vi "Host Image Acquisition Module.vi"(8 "error in":errorcluster, 11 "Operation":T3) -> (0 "error out":errorcluster, 1 "Image Acquired":bool, 2 "Acq In Progress":bool, 3 "Image":T2(plugin-control))   [LabVIEW 2013]
uses:
  Host Image Acquisition Module Enum.ctl
  Acquisition Settings Cluster.ctl
  <vilib>/vision/Image Controls.llb/IMAQ Image.ctl
  Image Acquisition Settings FG Enum.ctl
  System Status/Status FG Enum.ctl
  Image Processing/Mask ROI FG Enum.ctl
  <vilib>/rvi/interface/RandomDataEmulation/niFpgaWriteControlTemplate.vi
  <vilib>/rvi/interface/RandomDataEmulation/nirviRandomDataRunMethod.vi
  <vilib>/rvi/interface/RandomDataEmulation/nirviRandomDataDMAMethods.vi
  <vilib>/rvi/interface/RandomDataEmulation/niFpgaReadControlTemplate.vi
  Globals/Average Sector Data.vi
  <vilib>/rvi/interface/RandomDataEmulation/nirviRandomDataClose.vi
  <vilib>/rvi/interface/nirviReadWriteControl/nirviReadWriteControl.xnode
  FGs/FPGA_Reference.ctl
  Common/CL Configuration.ctl
  Common/CL Signal Mapping.ctl
  10-Tap 8-bit Camera without DRAM (FPGA-SIM).vi
  <vilib>/rvi/interface/nirviMethod/nirviMethod.xnode
  FPGA/Sector/Accumulate/Sector Parameter Cluster.ctl
  <vilib>/rvi/interface/nirviCloseFPGA/nirviCloseFPGA.xnode
  Common/Timing/Timing Lib.lvlib
  <vilib>/rvi/errors/niLvFpgaMergeErrorWithErrorCode.vi
panel:
  out "Actual Depth":u32
  out "Target Sim TO":bool
  out "Cam Data Timeout":bool
  out "Sector FIFO Timeout":bool
  out "Host DMA Timeout":bool
  out "Number of Elements to Write Host DMA":u32
  out "Number of Elements to Read Cam Data":u32
  out "Image Data":u64[](array[numeric])
  out "Elements Remaining":u32
  out "Words per image":u32
  out "Num Frames read":u32
  out "DMA Words per Image":u32
  out "Acquire":bool
  in  "Acquisition Settings Cluster":T1={"Image Width"=2040, "Image Height"=1088, "Frames To Acquire"=0, "Signal Mapping"=enum."Basler 10-tap", "DMA Buffer Size\n(In Images)"=64} {"Image Height" max=65535; "Image Width" max=65535 step=40}
  out "Buffer Size":u32
  out "Acq'd Frame Width":u32=2040
  out "DMA Write Timeout":bool
  in  "Start Serial Server":bool
  out "Frames Acq'd":u32=1
  out "Acq'd Frame Height":u32=1088
  out "Initialized":bool
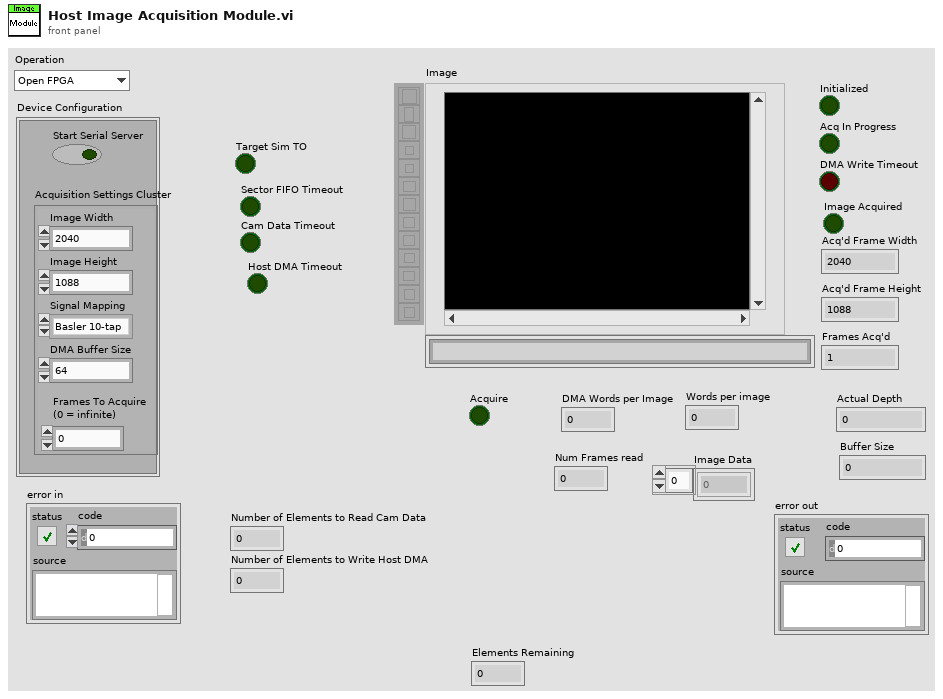
[diagram p1: front panel]
types:
  T1 = typedef "Acquisition Settings Cluster.ctl" = cluster{"Image Width":u32, "Image Height":u32, "Frames To Acquire":u32, "Signal Mapping":enum8{"Standard", "Basler 10-tap", "Vosskühler 10-tap"}, "DMA Buffer Size\n(In Images)":u32}
  T2 = typedef "IMAQ Image.ctl" = refnum<image>
  T3 = typedef "Host Image Acquisition Module Enum.ctl" = enum16{"Open FPGA", "Initialize DMA FIFO", "Load Sim Images", "Initialize Acquisition", "Update Sector Parameters", "Start Acquisition", "Aquire Image", "Read Averages", "Cancel Acquisition", "Close FPGA"}
  T4 = enum8{"Standard", "Basler 10-tap", "Vosskühler 10-tap"}
  T5 = typedef "Image Acquisition Settings FG Enum.ctl" = enum16{"Read", "Write"}
  T6 = typedef "Status FG Enum.ctl" = enum16{"Reset", "Read", "Write"}
  T7 = typedef "Mask ROI FG Enum.ctl" = enum16{"Read", "Write"}
  T8 = enum16{"big-endian, network order", "native, host order", "little-endian"}
  T9 = typedef "FPGA_Reference.ctl" = refnum<k20>
  T10 = typedef "Image Type" = u32
  T11 = typedef "Mask ROI Cluster.ctl" = cluster{"left annulus":T12, "right annulus":T12, "Threshold Range":cluster{"Lower value":dbl, "Upper value":dbl}, "[Avg BG]":u8[], "Number of Sectors":u8, "Left ROI":T13, "Right ROI":T13, "Left Start Angle Duty Cycle":fxp<+,8,0>, "Left End Angle Duty Cycle":fxp<+,8,0>, "Right End Angle Duty Cycle":fxp<+,8,0>, "Right Start Angle Duty Cycle":fxp<+,8,0>, "[Sector ROIs]":T13[]}
  T12 = typedef "IMAQ Circle" = cluster{"Center X":i32, "Center Y":i32, "Inner Radius":i32, "Outer Radius":i32, "Start Angle":dbl, "End Angle":dbl}
  T13 = typedef "ROI Descriptor" = cluster{"Global Rectangle":i32[], "Contours":cluster{"ID":enum32{"External", "Internal"}, "Type":u32, "Coordinates":i32[]}[]}
  T14 = typedef "Sector Parameter Cluster.ctl" = cluster{"Start Angle":fxp<+/-,17,2>, "End Angle":fxp<+,17,3>, "Inner Radius":u16, "Outter Radius":u16, "Hinge X":u16, "Hinge Y":u16, "NumWingSectors":u8}
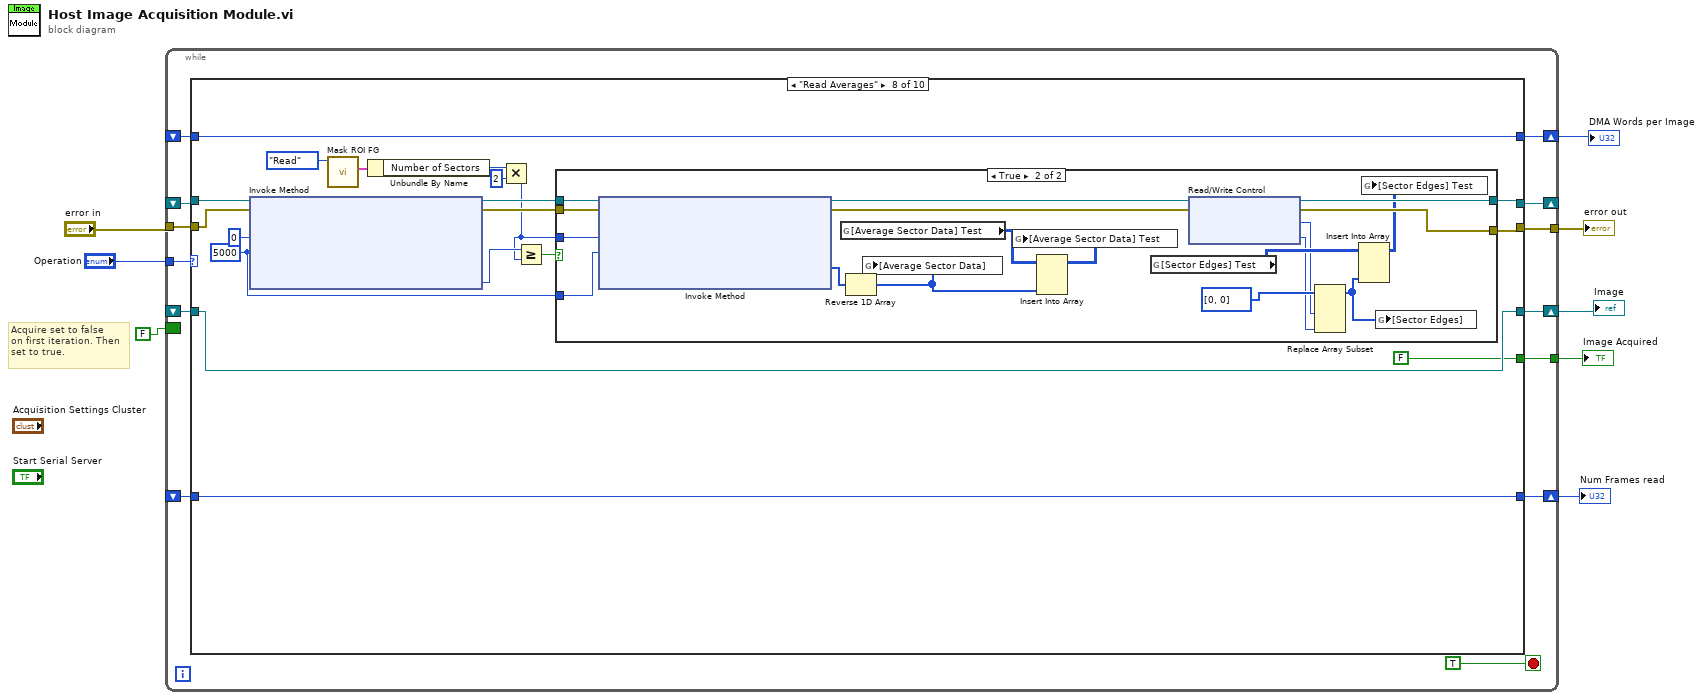
[diagram p0: block diagram]
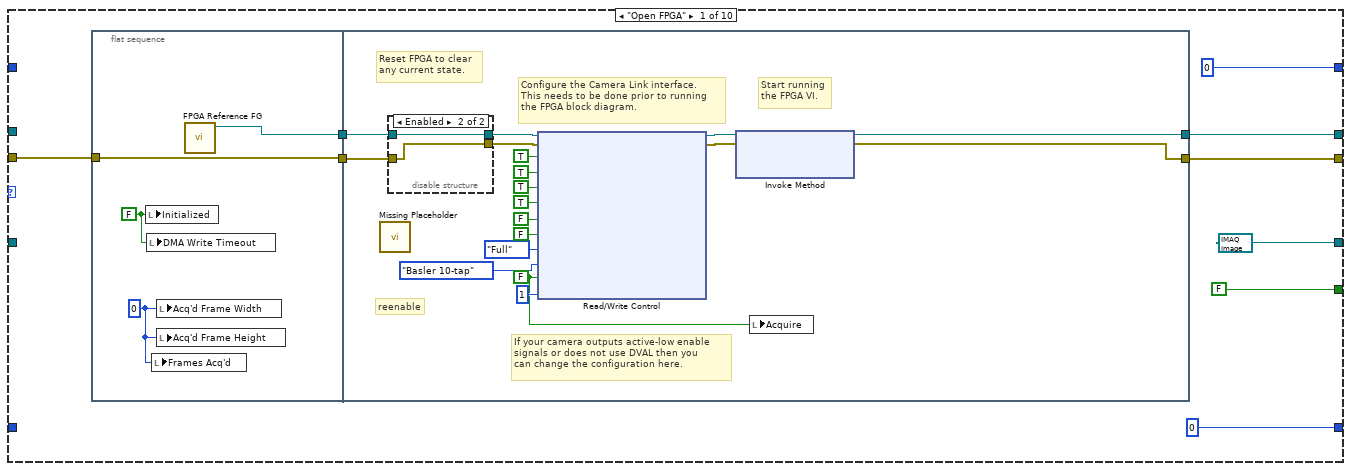
[diagram p2: hidden frame]
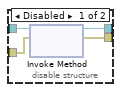
[diagram p3: hidden frame]
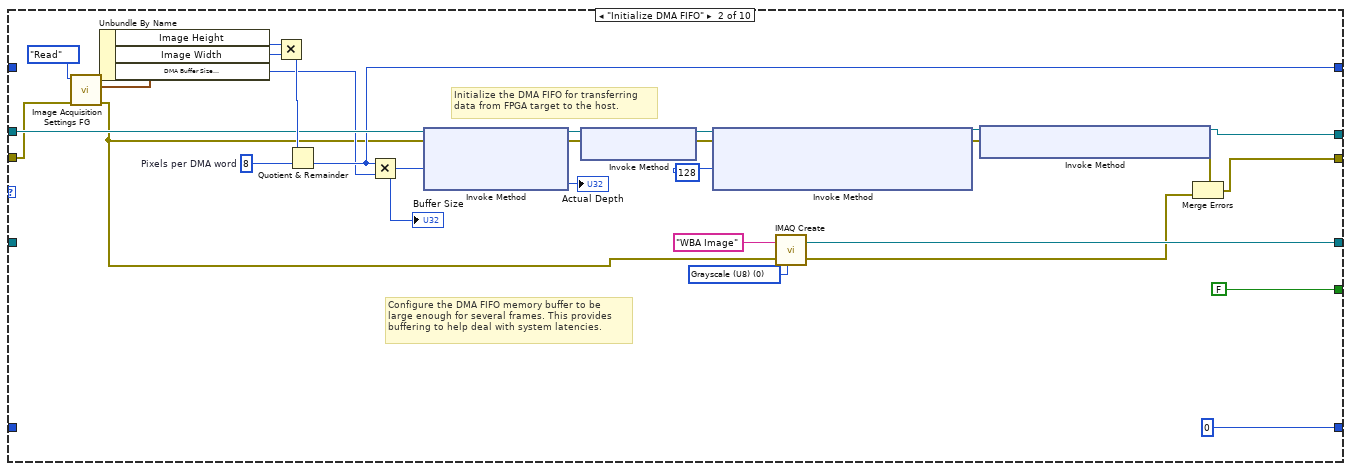
[diagram p4: hidden frame]
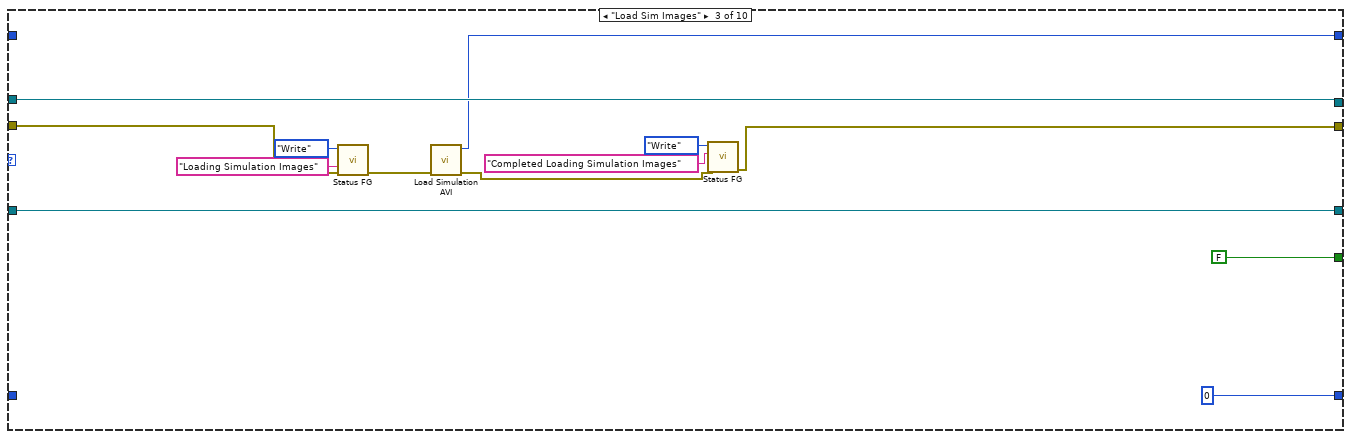
[diagram p5: hidden frame]
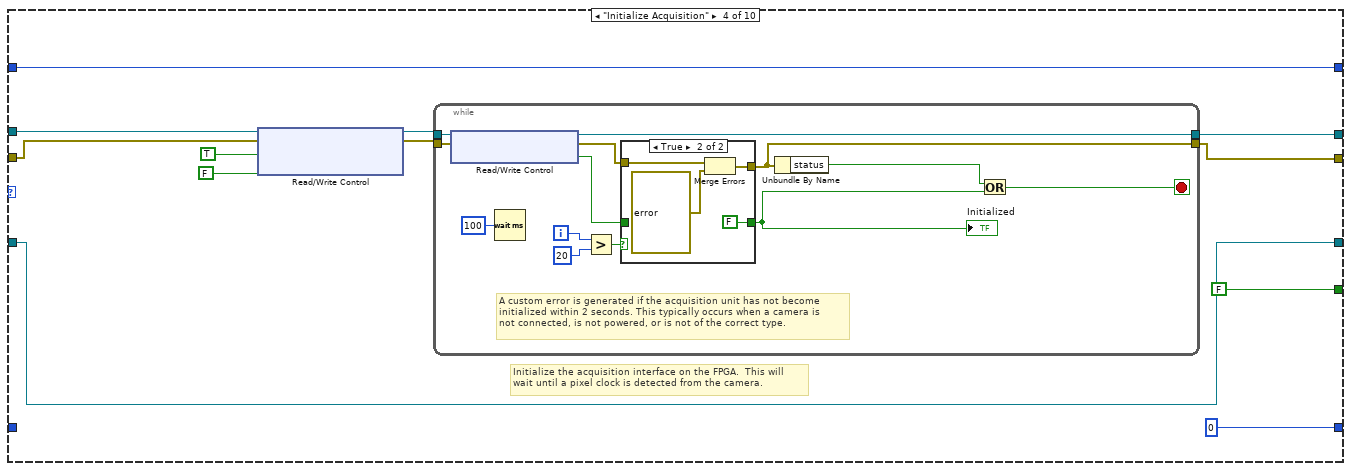
[diagram p6: hidden frame]
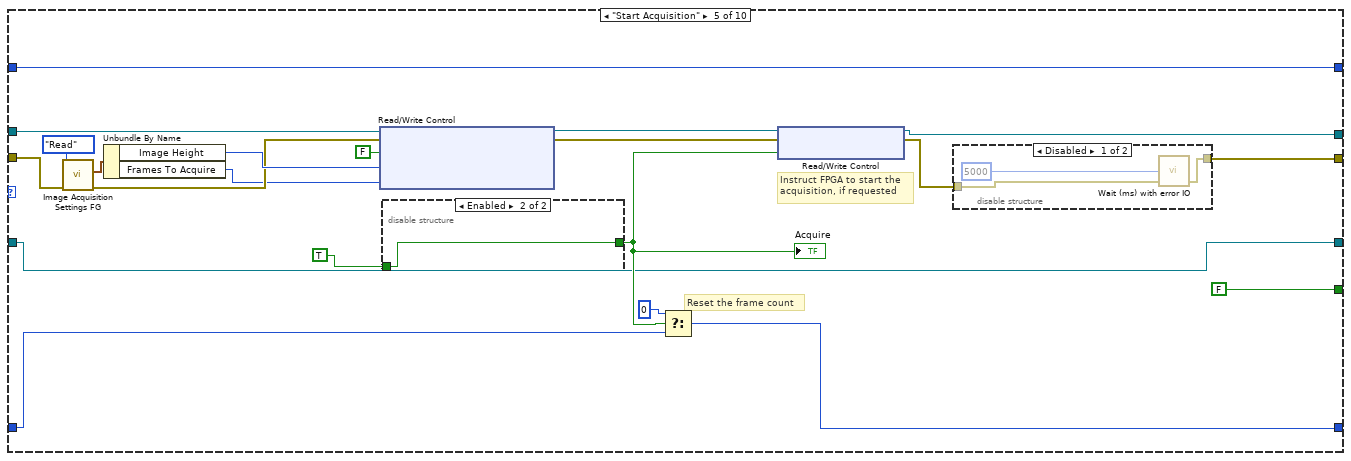
[diagram p8: hidden frame]
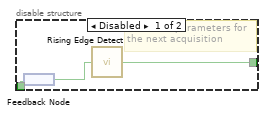
[diagram p10: hidden frame]
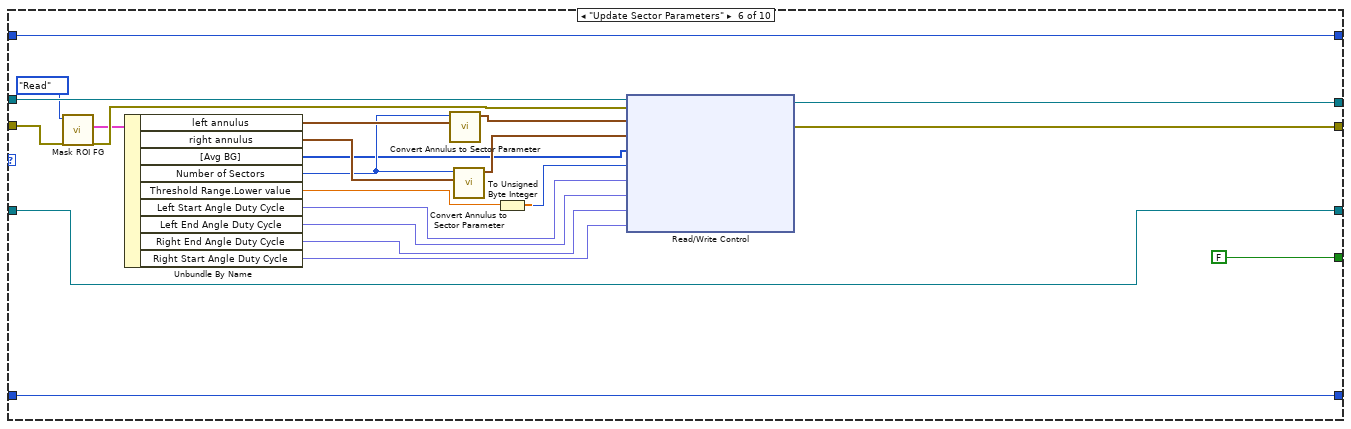
[diagram p11: hidden frame]
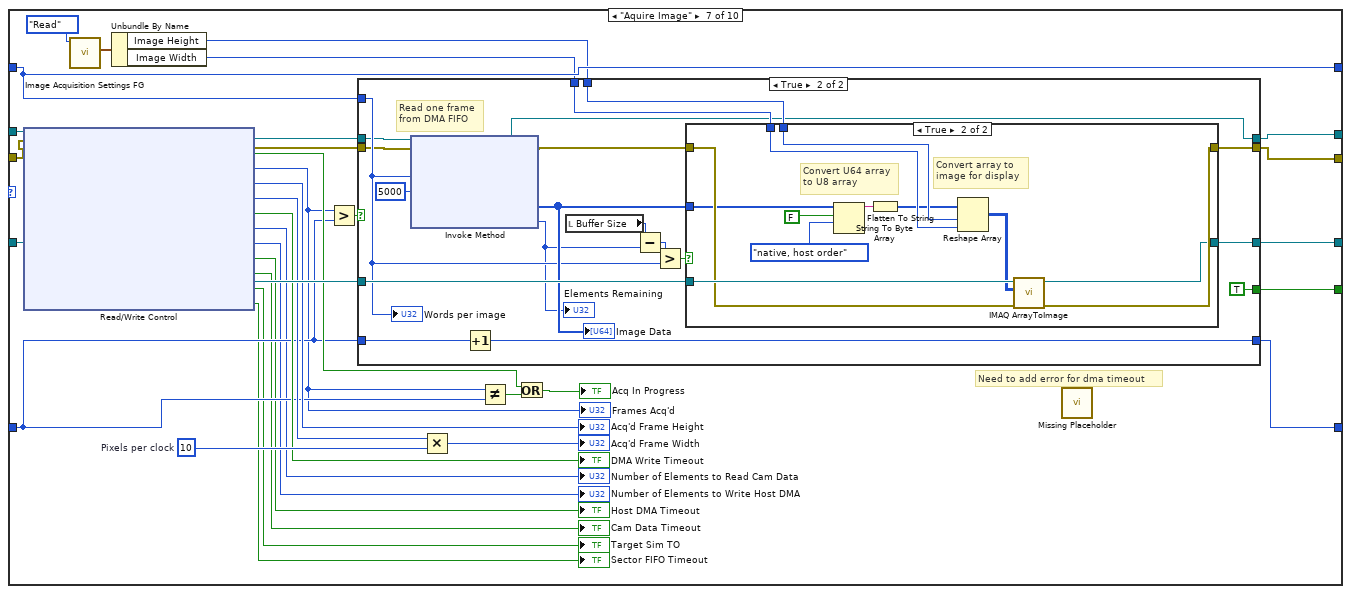
[diagram p12: hidden frame]
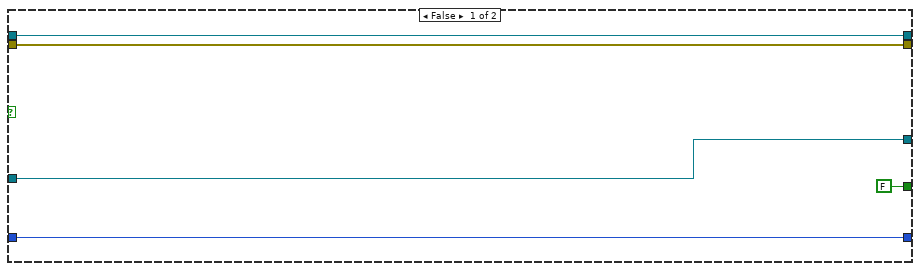
[diagram p13: hidden frame]
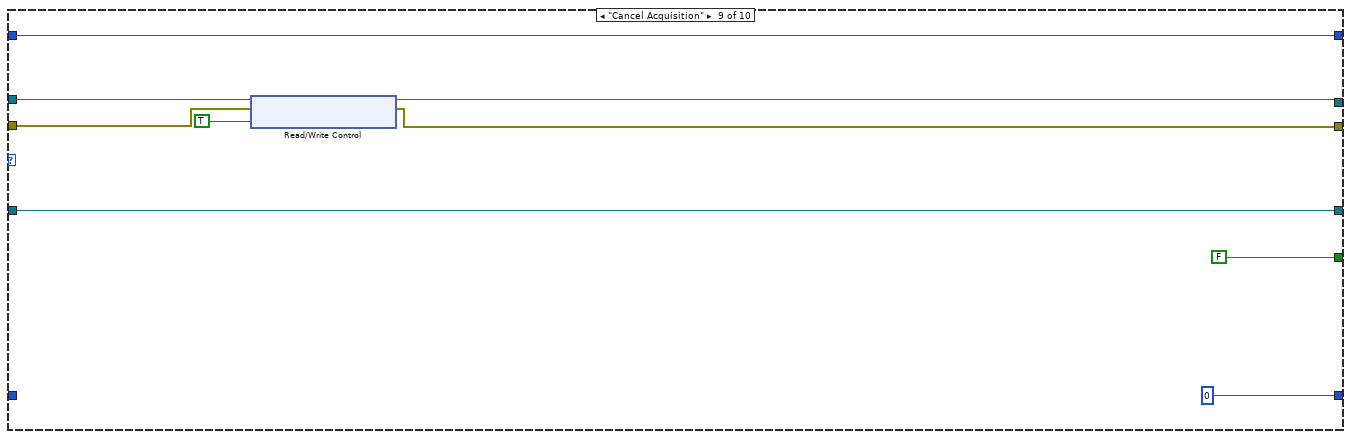
[diagram p16: hidden frame]
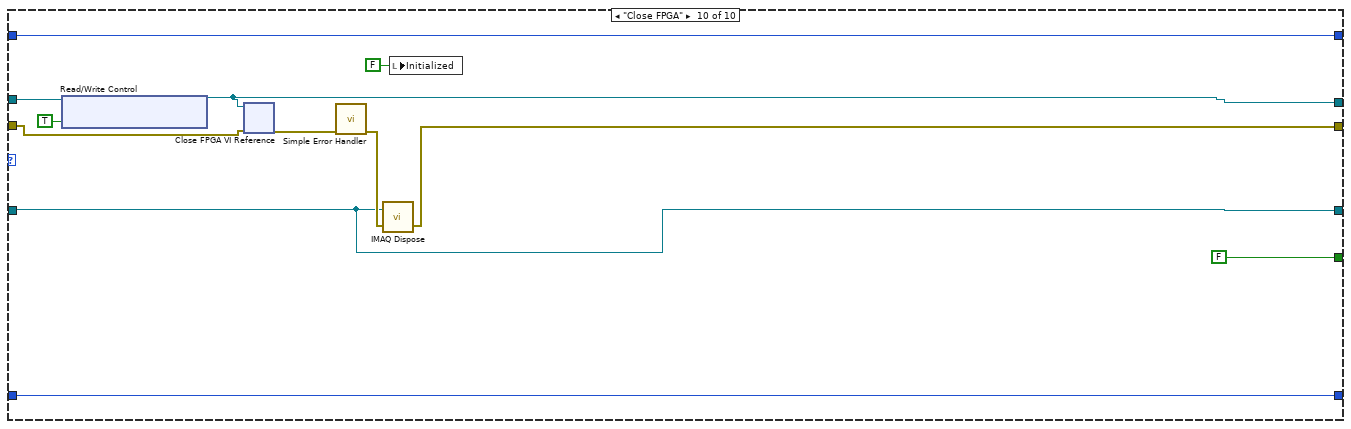
[diagram p17: hidden frame]
diagram:
  # "Acquire set to false\non first iteration. Then\nset to true."
  n1 = while {
    shift-right: [w20] -> _
    shift-left: _ -> [w16]
    tunnel: "error in" -> [w19]
    tunnel: "Operation" -> [w18]
    tunnel: [w17] -> w6
    shift-right: [w15] -> w3
    shift-left: _ -> [w14]
    shift-right: [w13] -> w4
    shift-left: _ -> [w10]
    shift-right: [w12] -> w2
    shift-left: _ -> [w11]
    border: FALSE ("Acquire") -> [_]
    tunnel: [w9] -> w1
    stop <- TRUE stop-if-true
    n2 = case shown="\"Read Averages\"" w18 {
      tunnel: w19 -> [w30 w74 w95 w102 w145 w181 w196 w265 w297 w303]
      tunnel: [w29 w66 w98 w108 w138 w177 w214 w271 w299 w304] -> w20
      tunnel: [w28 w67 w89 w104 w136 w178 w213 w266 w296 w310] -> w17
      tunnel: w16 -> [_ w82 w98 w109 w146 w183 w215 w272 w301 w306]
      tunnel: [u32 0 w81 w97 w107 w141 w182 w206 w270 w295 w307] -> w15
      tunnel: w14 -> [_ _ _ w107 w141 w182 w206 w270 w295 w307]
      tunnel: [T2 refnum ("New Image") w77 w99 w103 w140 w168 w208 w269 w298 w308] -> w13
      tunnel: [u32 0 u32 0 u32 0 u32 0 w142 w176 w212 w268 u32 0 w309] -> w12
      tunnel: w11 -> [_ _ _ _ w143 w176 w194 w268 _ w309]
      tunnel: w10 -> [_ _ w99 w103 w140 w168 w207 w269 w298 w308]
      tunnel: [FALSE ("Image Acquired") FALSE ("Image Acquired") FALSE ("Image Acquired") FALSE ("Image Acquired") FALSE ("Image Acquired") FALSE ("Image Acquired") w188 FALSE ("Image Acquired") FALSE ("Image Acquired") FALSE ("Image Acquired")] -> w9
      frame "Open FPGA" {
        n3 = flat-sequence {
          tunnel: w30 -> [w31]
          tunnel: [w32] -> w27
          tunnel: [w31] -> w26
          tunnel: [w37] -> w28
          tunnel: [w38] -> w29
          tunnel: w27 -> [w42]
          tunnel: w26 -> [w39]
          frame #0 {
            w33 = u32 0 ("Acq'd Frame Width")
            w34 = FALSE ("Initialized")
            n4 = local write "Initialized"(w34) -> ()
            n5 = local write "DMA Write Timeout"(w34) -> ()
            n6 = local write "Frames Acq'd"(w33) -> ()
            n7 = local write "Acq'd Frame Width"(w33) -> ()
            n8 = local write "Acq'd Frame Height"(w33) -> ()
            n9 = call "FPGA Reference FG.vi"() -> ("FPGA VI Reference Out"=w32:T9)  [unwired: 11 in]
          }
          frame #1 {
            w35 = FALSE ("Acq Control.Acquire")
            # "reenable"
            # "If your camera outputs active-low enable\nsignals or does not use DVAL then you \ncan change the configuration here."
            # "Start running\nthe FPGA VI."
            # "Reset FPGA to clear\nany current state."
            # "Configure the Camera Link interface.\nThis needs to be done prior to running\nthe FPGA block diagram."
            n10 = call "Missing Placeholder.vi"() -> ()  [unwired: 12 in]
            n11 = disable-structure shown="Enabled" {
              disable-tunnel: [w56 w58] -> w46
              disable-tunnel: [w55 w57] -> w44
              disable-tunnel: w42 -> [w54 w58]
              disable-tunnel: w39 -> [w53 w57]
              frame Disabled {
                n12 = xnode "Invoke Method"("FPGA VI Reference In"=w54, "error in"=w53) -> ("FPGA VI Reference Out"=w56:T9, "error out"=w55:errorcluster)
              }
              frame Enabled {
              }
            }
            n13 = xnode "Read/Write Control"("FPGA VI Reference In"=w46, "error in"=w44, "CL Config.FVAL Active High"=TRUE ("IO Module Config.CL FVAL Active High"), "CL Config.LVAL Active High"=TRUE ("IO Module Config.CL LVAL Active High"), "CL Config.DVAL Active High"=TRUE ("IO Module Config.CL DVAL Active High"), "CL Config.Spare Active High"=TRUE ("IO Module Config.CL Spare Active High"), "CL Config.Line Scan"=FALSE, "Acq Control.Ignore DVAL"=FALSE ("CL Config.Line Scan"), "CL Config.Configuration"=enum8{"Base", "Medium", "Full"}."Full", "CL Config.Signal Mapping"=T4."Basler 10-tap", "Acq Control.Acquire"=w35, "# of Frames to Average"=u8 1) -> ("FPGA VI Reference Out"=w43:T9, "error out"=w45:errorcluster)
            n14 = xnode "Invoke Method"("FPGA VI Reference In"=w43, "error in"=w45) -> ("FPGA VI Reference Out"=w38:T9, "error out"=w37:errorcluster)  [unwired: 1 in]
            n15 = local write "Acquire"(w35) -> ()
          }
        }
      }
      frame "Initialize DMA FIFO" {
        w78 = T10 0 items=["Grayscale (U8)", "Grayscale (I16)", "Grayscale (SGL)", "Complex (CSG)", "RGB (U32)", "HSL (U32)", "RGB (U64)", "Grayscale (U16)"] ("Image Type")
        w84 = u32 8  # Pixels per DMA word
        # "Configure the DMA FIFO memory buffer to be\nlarge enough for several frames. This provides\nbuffering to help deal with system latencies."
        # "Initialize the DMA FIFO for transferring\ndata from FPGA target to the host."
        n16 = call "Image Acquisition Settings FG.vi"("error in (no error)"=w74, "Operation"=Image_Acquisition_Settings_FG_Enum."Read") -> ("error out"=w69:errorcluster, "Acquisition Settings Out"=w75:T1)  [unwired: 8 in]
        n17 = Unbundle By Name(w75) -> ("Image Height"=w73:u32, "Image Width"=w72:u32, "DMA Buffer Size\n(In Images)"=w71:u32)
        n18 = Multiply(x=w73, y=w72) -> (x*y=w83:u32)
        n19 = Quotient & Remainder(x=w83, y=w84) -> (floor(x/y)=w81:u32)  [unwired: 1 out]
        n20 = Multiply(x=w81, y=w71) -> (x*y=w85:u32)
        "Buffer Size" <- w85
        n21 = xnode "Invoke Method"("FPGA VI Reference In"=w82, "error in"=w69, "Requested Depth"=w85) -> ("FPGA VI Reference Out"=w87:T9, "error out"=w86:errorcluster, "Actual Depth"=→"Actual Depth":u32)
        n22 = xnode "Invoke Method"("FPGA VI Reference In"=w87, "error in"=w86) -> ("FPGA VI Reference Out"=w64:T9, "error out"=w62:errorcluster)
        n23 = xnode "Invoke Method"("FPGA VI Reference In"=w64, "error in"=w62, "Requested Depth"=u32 128) -> ("FPGA VI Reference Out"=w61:T9, "error out"=w60:errorcluster)  [unwired: 1 out]
        n24 = call "IMAQ Create"("Image Name"="WBA Image", "Image Type"=w78, "error in (no error)"=w69) -> ("New Image"=w77:T2, "error out"=w68:errorcluster)  [unwired: 2 in]
        n25 = xnode "Invoke Method"("FPGA VI Reference In"=w61, "error in"=w60) -> ("FPGA VI Reference Out"=w66:T9, "error out"=w59:errorcluster)
        n26 = Merge Errors(w59, w68) -> (w67:errorcluster)
      }
      frame "Load Sim Images" {
        n27 = call "Status FG.vi"("error in (no error)"=w95, "Status In"="Loading Simulation Images", "Operation"=Status_FG_Enum."Write") -> ("error out"=w94:errorcluster)  [unwired: 7 in, 1 out]
        n28 = call "Load Simulation AVI.vi"("error in (no error)"=w94) -> ("error out"=w90:errorcluster, "Words per image"=w97:u32)  [unwired: 9 in]
        n29 = call "Status FG.vi"("error in (no error)"=w90, "Status In"="Completed Loading Simulation Images", "Operation"=Status_FG_Enum."Write") -> ("error out"=w89:errorcluster)  [unwired: 7 in, 1 out]
      }
      frame "Initialize Acquisition" {
        # "Initialize the acquisition interface on the FPGA.  This will\nwait until a pixel clock is detected from the camera."
        n30 = xnode "Read/Write Control"("FPGA VI Reference In"=w109, "error in"=w102, "Acq Control.Initialize"=TRUE ("Arm Acquisition"), "Acq Control.Cancel Acq"=FALSE) -> ("FPGA VI Reference Out"=w112:T9, "error out"=w111:errorcluster)
        n31 = while {
          tunnel: w112 -> [w121]
          tunnel: w111 -> [w120]
          tunnel: [w119] -> w108
          tunnel: [w122] -> w104
          i -> [w115]
          stop <- w125 stop-if-true
          # "A custom error is generated if the acquisition unit has not become\ninitialized within 2 seconds. This typically occurs when a camera is\nnot connected, is not powered, or is not of the correct type."
          n32 = xnode "Read/Write Control"("FPGA VI Reference In"=w121, "error in"=w120) -> ("FPGA VI Reference Out"=w119:T9, "error out"=w118:errorcluster, "Acq Status.Initialized"=w117:bool)
          n33 = Wait (ms)(milliseconds to wait=u32 100) -> ()  [unwired: 1 out]
          n34 = Greater?(x=w115, y=20) -> (0:w116:bool)
          n35 = case shown="True" w116 {
            tunnel: [w127 FALSE] -> w113
            tunnel: w117 -> [w127 _]
            tunnel: w118 -> [w126 w129]
            tunnel: [w126 w131] -> w122
            frame False {
            }
            frame True {
              n36 = Merge Errors(w129, errorcluster {"status"=TRUE, "code"=-8999, "source"="Acquisition Initialization: This error typically occurs when a camera is not properly connected, is not powered, or is not of the correct type."} ("error in")) -> (w131:errorcluster)
            }
          }
          "Initialized" <- w113
          n37 = Unbundle By Name(w122) -> ("status"=w124:bool)
          n38 = Or(x=w124, y=w113) -> (x .or. y?=w125:bool)
        }
      }
      frame "Start Acquisition" {
        # "Reset the frame count"
        # "Instruct FPGA to start the\nacquisition, if requested"
        n39 = call "Image Acquisition Settings FG.vi"("error in (no error)"=w145, "Operation"=Image_Acquisition_Settings_FG_Enum."Read") -> ("error out"=w144:errorcluster, "Acquisition Settings Out"=w152:T1)  [unwired: 8 in]
        n40 = Unbundle By Name(w152) -> ("Image Height"=w147:u32, "Frames To Acquire"=w134:u32)
        n41 = xnode "Read/Write Control"("FPGA VI Reference In"=w146, "error in"=w144, "Acq Control.Cancel Acq"=FALSE, "Acq Control.Line Scan Height"=w147, "Acq Control.Frames To Acq"=w134) -> ("FPGA VI Reference Out"=w132:T9, "error out"=w133:errorcluster)
        n42 = disable-structure shown="Enabled" {
          disable-tunnel: [w159 w160] -> w149
          disable-tunnel: TRUE ("Acquire") -> [w157 w160]
          frame Disabled {
            # "Write the parameters for\nthe next acquisition"
            n43 = feedback #1() -> (w158:bool)
            n44 = feedback-in #1(w157) -> ()
            n45 = call "Rising Edge Detect.vi"("Input"=w158) -> ("Pulse"=w159:bool)  [unwired: 4 in]
          }
          frame Enabled {
          }
        }
        "Acquire" <- w149
        n46 = Select(t=u32 0, s=w149, f=w143) -> (s? t:f=w142:u32)
        n47 = xnode "Read/Write Control"("FPGA VI Reference In"=w132, "error in"=w133, "Acq Control.Acquire"=w149) -> ("FPGA VI Reference Out"=w138:T9, "error out"=w137:errorcluster)
        n48 = disable-structure shown="Disabled" {
          disable-tunnel: w137 -> [w154 w156]
          disable-tunnel: [w153 w156] -> w136
          frame Disabled {
            n49 = call "Wait (ms) with error IO.vi"("error in (no error)"=w154, "milliseconds to wait"=u32 5000) -> ("error out"=w153:errorcluster)  [unwired: 3 in]
          }
          frame Enabled {
          }
        }
      }
      frame "Update Sector Parameters" {
        n50 = call "Mask ROI FG.vi"("error in (no error)"=w181, "Operation"=Mask_ROI_FG_Enum."Read") -> ("error out"=w180:errorcluster, "Mask ROI Out"=w175:T11)  [unwired: 8 in]
        n51 = Unbundle By Name(w175) -> ("left annulus"=w174:T12, "right annulus"=w172:T12, "[Avg BG]"=w169:u8[], "Number of Sectors"=w171:u8, "Threshold Range.Lower value"=w166:dbl, "Left Start Angle Duty Cycle"=w164:fxp<+,8,0>, "Left End Angle Duty Cycle"=w163:fxp<+,8,0>, "Right End Angle Duty Cycle"=w162:fxp<+,8,0>, "Right Start Angle Duty Cycle"=w161:fxp<+,8,0>)
        n52 = call "Convert Annulus to Sector Parameter.vi"("Annulus"=w174, "NumWingSectors"=w171) -> ("Sector Parameter"=w173:T14)  [unwired: 9 in]
        n53 = call "Convert Annulus to Sector Parameter.vi"("Annulus"=w172, "NumWingSectors"=w171) -> ("Sector Parameter"=w170:T14)  [unwired: 9 in]
        n54 = To Unsigned Byte Integer(number=w166) -> (unsigned 8bit integer=w165:u8)
        n55 = xnode "Read/Write Control"("FPGA VI Reference In"=w183, "error in"=w180, "Sector Parameters Left"=w173, "Sector Parameters Right"=w170, "[Average BG Intensity]"=w169, "Sector Threshold"=w165, "Left Start Angle Duty Cycle"=w164, "Left End Angle Duty Cycle"=w163, "Right End Angle Duty Cycle"=w162, "Right Start Angle Duty Cycle"=w161) -> ("FPGA VI Reference Out"=w177:T9, "error out"=w178:errorcluster)
      }
      frame "Aquire Image" {
        w204 = u32 10  # Pixels per clock
        # "Need to add error for dma timeout"
        n56 = xnode "Read/Write Control"("FPGA VI Reference In"=w215, "error in"=w196) -> ("FPGA VI Reference Out"=w211:T9, "error out"=w210:errorcluster, "Acq Status.Acq In Progress"=w195:bool, "Acq Status.Frames Acq'd"=w193:u32, "Acq Status.Lines Per Frame"=→"Acq'd Frame Height":u32, "Acq Status.Clocks Per Line"=w203:u32, "Acq Status.DMA Write Timeout"=→"DMA Write Timeout":bool, "Number of Elements to Read Cam Data"=→"Number of Elements to Read Cam Data":u32, "Number of Elements to Write Host DMA"=→"Number of Elements to Write Host DMA":u32, "Host DMA Timeout"=→"Host DMA Timeout":bool, "Cam Data Timeout"=→"Cam Data Timeout":bool, "Target Sim TO"=→"Target Sim TO":bool, "Sector FIFO Timeout"=→"Sector FIFO Timeout":bool)
        "Frames Acq'd" <- w193
        n57 = call "Image Acquisition Settings FG.vi"("Operation"=Image_Acquisition_Settings_FG_Enum."Read") -> ("Acquisition Settings Out"=w199:T1)  [unwired: 9 in, 1 out]
        n58 = Unbundle By Name(w199) -> ("Image Height"=w198:u32, "Image Width"=w197:u32)
        n59 = Greater?(x=w193, y=w194) -> (0:w209:bool)
        n60 = case shown="True" w209 {
          tunnel: w211 -> [w219 w222]
          tunnel: w210 -> [w218 w223]
          tunnel: w198 -> [_ w239]
          tunnel: w197 -> [_ w238]
          tunnel: w207 -> [w220 w237]
          tunnel: [w218 w235] -> w213
          tunnel: [w219 w234] -> w214
          tunnel: w194 -> [w217 w233]
          tunnel: [w217 w232] -> w212
          tunnel: w206 -> [_ w229]
          tunnel: [w220 w228] -> w208
          tunnel: [FALSE ("Image Acquired") TRUE ("Image Acquired")] -> w188
          frame False {
          }
          frame True {
            # "Read one frame\nfrom DMA FIFO"
            n61 = xnode "Invoke Method"("FPGA VI Reference In"=w222, "error in"=w223, "Number of Elements"=w229, "Timeout (ms)"=5000) -> ("FPGA VI Reference Out"=w234:T9, "error out"=w236:errorcluster, "Data"=w231:u64[], "Elements Remaining"=w226:u32)
            "Elements Remaining" <- w226
            "Image Data" <- w231
            n62 = Increment(x=w233) -> (x+1=w232:u32)
            n63 = local read "Buffer Size"() -> (w227:u32)
            n64 = Subtract(x=w227, y=w226) -> (x-y=w225:u32)
            n65 = Greater?(x=w225, y=w229) -> (0:w230:bool)
            n66 = case shown="True" w230 {
              tunnel: w239 -> [_ w253]
              tunnel: w238 -> [_ w252]
              tunnel: w237 -> [w240 w251]
              tunnel: w236 -> [w241 w250]
              tunnel: [w241 w249] -> w235
              tunnel: w231 -> [_ w246]
              tunnel: [w240 w242] -> w228
              frame False {
                # "Do not display the image if we're\nfalling behind in the acquisition."
              }
              frame True {
                # "Convert U64 array\nto U8 array"
                # "Convert array to\nimage for display"
                n67 = Flatten To String(anything=w246, prepend array or string size? (T)=FALSE, byte order (0:big-endian, network order)=T8."native, host order") -> (data string=w244:string)  [unwired: 1 in, 2 out]
                n68 = String To Byte Array(string=w244) -> (unsigned byte array=w243:u8[])
                n69 = Reshape Array(w243, w253, w252) -> (w248:u8[][])
                n70 = call "IMAQ ArrayToImage"("error in (no error)"=w250, "Image Pixels (U8)"=w248, "Image"=w251) -> ("error out"=w249:errorcluster, "Image Out"=w242:T2)  [unwired: 7 in]
              }
            }
            "Words per image" <- w229
          }
        }
        n71 = Multiply(x=w203, y=w204) -> (x*y=→"Acq'd Frame Width":u32)
        n72 = Not Equal?(x=w193, y=w194) -> (x != y?=w192:bool)
        n73 = Or(x=w195, y=w192) -> (x .or. y?=→"Acq In Progress":bool)
        n74 = call "Missing Placeholder.vi"() -> ()  [unwired: 12 in]
      }
      frame "Read Averages" {
        w261 = 5000 ("Timeout (ms)")
        n75 = xnode "Invoke Method"("FPGA VI Reference In"=w272, "error in"=w265, "Number of Elements"=u32 0, "Timeout (ms)"=w261) -> ("FPGA VI Reference Out"=w263:T9, "error out"=w262:errorcluster, "Elements Remaining"=w256:u32)  [unwired: 1 out]
        n76 = call "Mask ROI FG.vi"("Operation"=Mask_ROI_FG_Enum."Read") -> ("Mask ROI Out"=w259:T11)  [unwired: 9 in, 1 out]
        n77 = Unbundle By Name(w259) -> ("Number of Sectors"=w257:u8)
        n78 = Multiply(x=w257, y=u8 2) -> (x*y=w255:u8)
        n79 = Greater Or Equal?(x=w256, y=w255) -> (x >= y?=w258:bool)
        n80 = case shown="True" w258 {
          tunnel: w263 -> [w274 w292]
          tunnel: w262 -> [w273 w291]
          tunnel: w261 -> [_ w290]
          tunnel: [w274 w283] -> w271
          tunnel: [w273 w284] -> w266
          tunnel: w255 -> [_ w289]
          frame False {
          }
          frame True {
            n81 = xnode "Invoke Method"("FPGA VI Reference In"=w292, "error in"=w291, "Number of Elements"=w289, "Timeout (ms)"=w290) -> ("FPGA VI Reference Out"=w286:T9, "error out"=w285:errorcluster, "Data"=w280:u8[])  [unwired: 1 out]
            n82 = global read "Average Sector Data.vi" "[Average Sector Data] Test"() -> (w288:u8[][])
            n83 = Reverse 1D Array(array=w280) -> (reversed array=w279:u8[])
            n84 = global write "Average Sector Data.vi" "[Average Sector Data]"(w279) -> ()
            n85 = Insert Into Array(array=w288, new element=w279) -> (w287:u8[][])  [unwired: 2 in]
            n86 = global write "Average Sector Data.vi" "[Average Sector Data] Test"(w287) -> ()
            n87 = global read "Average Sector Data.vi" "[Sector Edges] Test"() -> (w282:u8[][])
            n88 = xnode "Read/Write Control"("FPGA VI Reference In"=w286, "error in"=w285) -> ("FPGA VI Reference Out"=w283:T9, "error out"=w284:errorcluster, "Right Sector Edge"=w277:u8, "Left Sector Edge"=w276:u8)
            n89 = Replace Array Subset(array=u8[] [0, 0] ("[Sector Edges]"), new element #1=w277, new element #2=w276) -> (w275:u8[])  [unwired: 2 in]
            n90 = Insert Into Array(array=w282, new element=w275) -> (w281:u8[][])  [unwired: 2 in]
            n91 = global write "Average Sector Data.vi" "[Sector Edges] Test"(w281) -> ()
            n92 = global write "Average Sector Data.vi" "[Sector Edges]"(w275) -> ()
          }
        }
      }
      frame "Cancel Acquisition" {
        n93 = xnode "Read/Write Control"("FPGA VI Reference In"=w301, "error in"=w297, "Acq Control.Cancel Acq"=TRUE) -> ("FPGA VI Reference Out"=w299:T9, "error out"=w296:errorcluster)
      }
      frame "Close FPGA" {
        n94 = xnode "Read/Write Control"("FPGA VI Reference In"=w306, "Acq Control.Cancel Acq"=TRUE) -> ("FPGA VI Reference Out"=w304:T9)  [unwired: 1 in, 1 out]
        n95 = xnode "Close FPGA VI Reference"("FPGA VI Reference In"=w304, "error in"=w303) -> ("error out"=w313:errorcluster)
        n96 = call <vilib>:"Simple Error Handler.vi"("error in (no error)"=w313) -> ("error out"=w311:errorcluster)  [unwired: 4 in, 4 out]
        n97 = call "IMAQ Dispose"("Image"=w308, "error in (no error)"=w311) -> ("error out"=w310:errorcluster)  [unwired: 4 in]
        n98 = local write "Initialized"(FALSE ("Initialized")) -> ()
      }
    }
  }
  "error out" <- w6
  "Image" <- w4
  "DMA Words per Image" <- w3
  "Num Frames read" <- w2
  "Image Acquired" <- w1
